vi "Test A.vi"(8 "error in (no error)":errorcluster) -> (0 "error out":errorcluster)   [LabVIEW 2019, in "Simple Example(Station1).lvlib"]
uses:
  Simple Example(Station1).lvlib
  d31799f9-9e59-4a03-9ea0-60b3ce935fd9.vi
  00355e06-9aa9-4587-985a-8f165454d30f.vi
  Read Limit(Double Float).vi
  LVUT Global 1.vi
  <vilib>/Utility/Data Type/Get Type Information.vi
  Almost Equal.vi
  Unit Test Engine Tools.lvlib
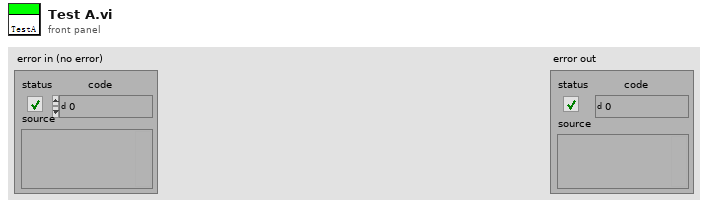
[diagram p1: front panel]
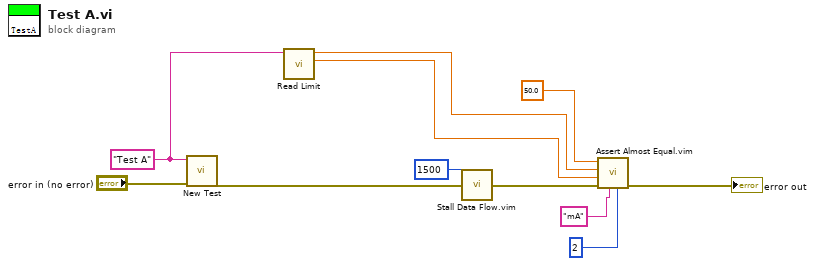
[diagram p0: block diagram]
diagram:
  w1 = "Test A" ("Test")
  n1 = call "New Test.vi"("error in (no error)"="error in (no error)", "Test"=w1) -> ("error out"=w10:errorcluster)  [unwired: 9 in]
  n2 = call-poly "Read Limit.vi"("Test"=w1) -> ("a"=w2:dbl, "b"=w3:dbl)  [unwired: 9 in]
  n3 = call "Stall Data Flow.vim"("value in"=w10, "milliseconds to wait"=u32 1500) -> ("value out"=w8:errorcluster)  [unwired: 1 out]
  n4 = call "Assert Almost Equal.vim"("precision (2)"=i16 2 ("precision (6)"), "Unit"="mA", "error in (no error)"=w8, "a"=w2, "b"=w3, "x"=50.0 ("X")) -> ("error out"=→"error out":errorcluster)  [unwired: 5 in]
